vi "RT_Angle_Of_Attack_in_DLR_Navigation_Reference_System (SubVI).vi"(8 "i":i32, 9 "V_wind [m/s]":dbl[][](array[numeric]), 10 "V (m/s)":dbl[](array[numeric]), 11 "DCM":dbl[][](array[numeric])) -> (2 "AoA_yaw (rad)":dbl, 3 "AoA_pitch (rad)":dbl)   [LabVIEW 2011]
uses:
  <vilib>/Analysis/Matrix/Datatypes/RealMatrix.ctl
  <vilib>/Analysis/Matrix/Numeric/Conversions/Array To Matrix - RA2.vi
  <vilib>/Analysis/baseanly.llb/Real A x B.vi
  <vilib>/Analysis/Matrix/Numeric/Conversions/Matrix To Array - RM.vi
  <vilib>/Analysis/NI_AALBase.lvlib
  <vilib>/Analysis/Matrix/NI_Matrix.lvlib
panel:
  out "r":dbl[](array[numeric])
  out "v":dbl[](array[numeric])
  out "r_matrix":T1
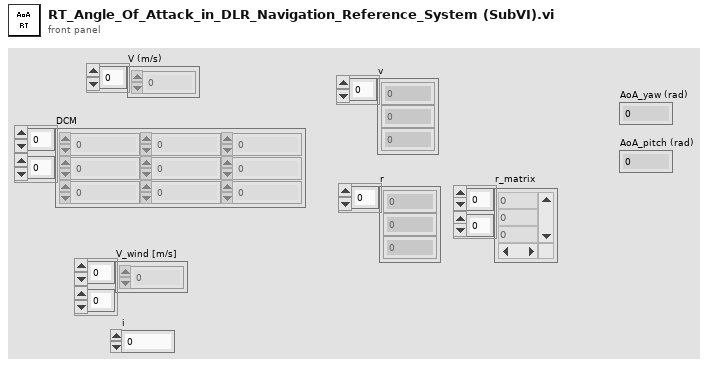
[diagram p1: front panel]
types:
  T1 = typedef "NI_Matrix.lvlib/RealMatrix.ctl" = dbl[][]
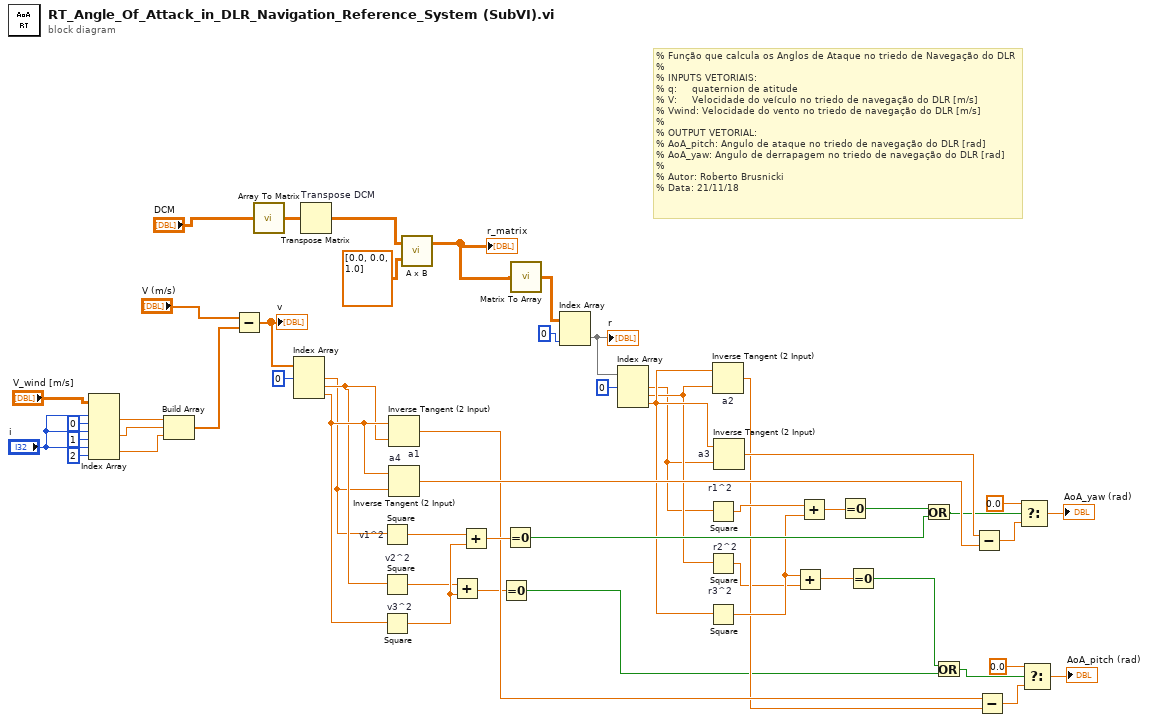
[diagram p0: block diagram]
diagram:
  # "% Função que calcula os Anglos de Ataque no triedo de Navegação do DLR \n%\n% INPUTS VETORIAIS: \n% q:     quaternion de atitude   \n% V:     Velocidade do veículo no triedo de navegação do DLR [m/s]\n% Vwind: Velocidade do vento no triedo de navegação do DLR [m/s]\n%\n% OUTPUT VETORIAL:\n% AoA_pitch: Angulo de ataque no triedo de navegação do DLR [rad]\n% AoA_yaw: Angulo de derrapagem no triedo de navegação do DLR [rad]\n%\n% Autor: Roberto Brusnicki\n% Data: 21/11/18"
  n1 = Index Array(array="V_wind [m/s]", index (row) #1="i", index (col) #1=0 ("disabled index (col)"), index (row) #2="i", index (col) #2=1 ("disabled index (col)"), index (row) #3="i", index (col) #3=2 ("disabled index (col)")) -> (element #1=w4:dbl, element #2=w3:dbl, element #3=w2:dbl)
  n2 = Build Array(w4, w3, w2) -> (w1:dbl[])
  n3 = Subtract(x="V (m/s)", y=w1) -> (x-y=w21:dbl[])
  "v" <- w21
  n4 = call-poly <vilib>:"Array To Matrix.vi"("Real 2D Array"="DCM") -> ("Real Matrix"=w14:T1)
  n5 = Index Array(array=w21, index #1=0 ("index (row)")) -> (element #1=w22:dbl, element #2=w23:dbl, element #3=w24:dbl)  [unwired: 2 in]
  n6 = Transpose Matrix "Transpose DCM"(1:w14) -> (0:w15:T1)
  n7 = Square "v1^2"(x=w22) -> (x^2=w40:dbl)
  n8 = Square "v2^2"(x=w23) -> (x^2=w28:dbl)
  n9 = Square "v3^2"(x=w24) -> (x^2=w41:dbl)
  n10 = Inverse Tangent (2 Input) "a1"(1:w23, 2:w24) -> (0:w37:dbl)
  n11 = Inverse Tangent (2 Input) "a4"(1:w22, 2:w24) -> (0:w52:dbl)
  n12 = call-poly <vilib>:"A x B.vi"("B"=T1 [[0.0], [0.0], [1.0]], "A"=w15) -> ("A x B"=w12:T1)  [unwired: 1 out]
  "r_matrix" <- w12
  n13 = Add(x=w28, y=w41) -> (x+y=w31:dbl)
  n14 = Add(x=w40, y=w41) -> (x+y=w42:dbl)
  n15 = Equal To 0?(x=w31) -> (x = 0?=w33:bool)
  n16 = Equal To 0?(x=w42) -> (x = 0?=w46:bool)
  n17 = call-poly <vilib>:"Matrix To Array.vi"("Real Matrix"=w12) -> ("Real 2D Array"=w17:dbl[][])
  n18 = Index Array(array=w17, index (col)=0 ("index (row)")) -> (element=w19:dbl[])  [unwired: 1 in]
  "r" <- w19
  n19 = Index Array(array=w19, index #1=0 ("index (row)")) -> (element #1=w25:dbl, element #2=w26:dbl, element #3=w27:dbl)  [unwired: 2 in]
  n20 = Square "r1^2"(x=w25) -> (x^2=w43:dbl)
  n21 = Square "r2^2"(x=w26) -> (x^2=w29:dbl)
  n22 = Square "r3^2"(x=w27) -> (x^2=w44:dbl)
  n23 = Inverse Tangent (2 Input) "a2"(1:w26, 2:w27) -> (0:w36:dbl)
  n24 = Inverse Tangent (2 Input) "a3"(1:w25, 2:w27) -> (0:w53:dbl)
  n25 = Add(x=w44, y=w29) -> (x+y=w30:dbl)
  n26 = Add(x=w43, y=w44) -> (x+y=w45:dbl)
  n27 = Equal To 0?(x=w45) -> (x = 0?=w47:bool)
  n28 = Equal To 0?(x=w30) -> (x = 0?=w32:bool)
  n29 = Or(x=w47, y=w46) -> (x .or. y?=w51:bool)
  n30 = Or(x=w32, y=w33) -> (x .or. y?=w34:bool)
  n31 = Subtract(x=w53, y=w52) -> (x-y=w49:dbl)
  n32 = Subtract(x=w37, y=w36) -> (x-y=w38:dbl)
  n33 = Select(t=0.0, s=w51, f=w49) -> (s? t:f=→"AoA_yaw (rad)":dbl)
  n34 = Select(t=0.0, s=w34, f=w38) -> (s? t:f=→"AoA_pitch (rad)":dbl)
